vi "ClsGeometryPeakSignal(thicknessandpeak)IDmakerforCHRocodileII.vi"(0 "Peak Signal Name":i32(ring) items=["PeakValue"=0, "PeakValue Median"=4, "PeakWidth"=5], 1 "Peak Index(no more than 4 for multiple channel devices)":i32(ring) items=["0", "1", "2", "3", "4", "5", "6", "7", "8", "9", "10", "11", "12", "13", "14", "15"], 2 "Combination(peak or thickness)":i32(ring) items=["Peak", "Thickness"], 3 "Statistics for a given\naveraging period\n(set by AVD):":i32(ring) items=["Average"=0, "Standard Deviation"=1, "Minimum"=3, "Maximum"=4, "Peak-to-peak (max-min)"=5], 4 "Value Encoding(Geometric: distance and thickness)":i32(ring)) -> (5 "Peak Signal ID":i32)   [LabVIEW 2015]
doc: "Geometry Peak Signal (thickness and peak) ID maker(for CHRocodile 2 Signal/Multi Channel devices):\n\nGenerate the signal ID for a geometric peak signal. For multiple channel devices, peak signals are those who appear once each channel each sample(for example, one sample in a 192-channel devices can contain only one certain global signal such as the sample counter but can contain 192 peak signals (one for each channel) such as the peak value). Geometry signals are those who should have a unit of distance. Geometry signals include distances and thickness. Non geometric peak signals are those without a distance unit, examples of which include the peak intensity/quality, the CCD position, etc..\n\nPeak Signal Name[Input]: the peak signal name.\n\nPeak Index[Input]: the index of peak of which data is acquired. $NOP will set the maximum amount of peaks available. The index of peak starts from 0.\n\nCombination[Input]; whether a peak or a thickness(combination of two peaks) is read.\n\nStatistics[Input]: the statistics for a given averaging period(set by AVD).\n\nValue Encoding(Nongeometric)[Input]: the encoding method for the signal for the nongeometric signals.\n\nNon-geometric peak signal ID[Output]: the calculated non-geometric peak signal ID."
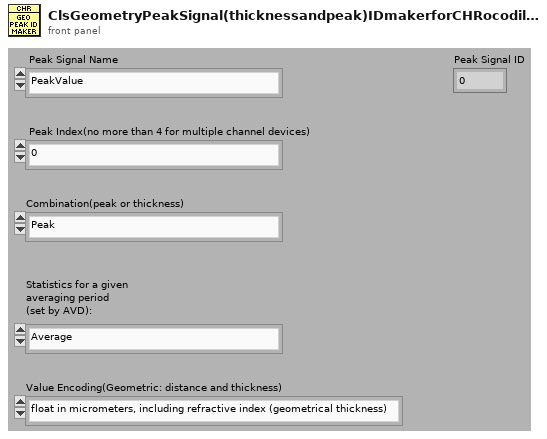
[diagram p1: front panel]
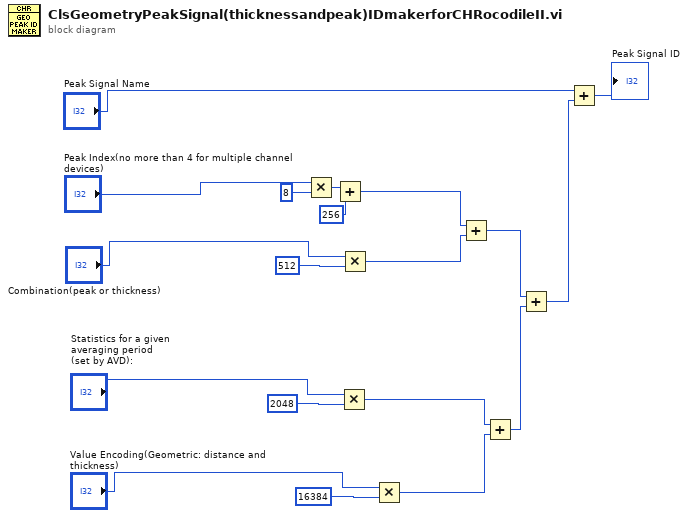
[diagram p0: block diagram]
diagram:
  n1 = Multiply(x="Peak Index(no more than 4 for multiple channel devices)", y=8) -> (x*y=w3:i32)
  n2 = Add(x=w3, y=256) -> (x+y=w11:i32)
  n3 = Multiply(x="Statistics for a given\naveraging period\n(set by AVD):", y=2048) -> (x*y=w13:i32)
  n4 = Multiply(x="Combination(peak or thickness)", y=512) -> (x*y=w12:i32)
  n5 = Multiply(x="Value Encoding(Geometric: distance and thickness)", y=16384) -> (x*y=w14:i32)
  n6 = Add(x=w11, y=w12) -> (x+y=w15:i32)
  n7 = Add(x=w13, y=w14) -> (x+y=w16:i32)
  n8 = Add(x=w15, y=w16) -> (x+y=w18:i32)
  n9 = Add(x="Peak Signal Name", y=w18) -> (x+y=→"Peak Signal ID":i32)
